vi "test.vi"() -> ()   [LabVIEW 2019]
uses:
  Valve_class/Valve.lvclass
panel:
  out "error out":errorcluster
  in  "VISA resource name":refnum<visa-resource-name>
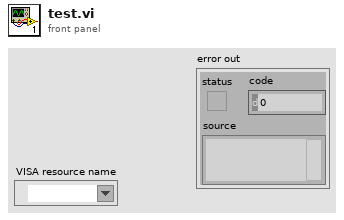
[diagram p1: front panel]
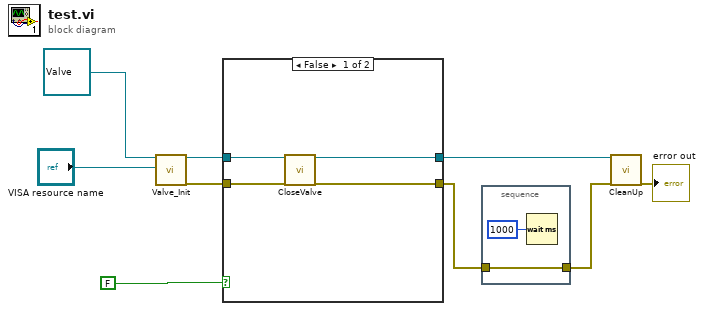
[diagram p0: block diagram]
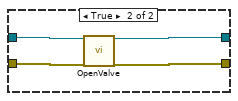
[diagram p2: hidden frame]
diagram:
  n1 = call "Valve_Init.vi"("object in"=refnum<class "Valve.lvclass"> refnum, "VISA resource name"="VISA resource name") -> ("object out"=w9:refnum<class "Valve.lvclass">, "error out"=w8:errorcluster)  [unwired: 16 in]
  n2 = case shown="False" FALSE {
    tunnel: w9 -> [w13 w17]
    tunnel: w8 -> [w11 w16]
    tunnel: [w12 w15] -> w5
    tunnel: [w10 w14] -> w4
    frame False {
      n3 = call-dynamic "CloseValve.vi"("object in"=w13, "error in (no error)"=w11) -> ("object out"=w12:refnum<class "Valve.lvclass">, "error out"=w10:errorcluster)  [unwired: 16 in]
    }
    frame True {
      n4 = call-dynamic "OpenValve.vi"("object in"=w17, "error in (no error)"=w16) -> ("object out"=w15:refnum<class "Valve.lvclass">, "error out"=w14:errorcluster)  [unwired: 16 in]
    }
  }
  n5 = stacked-sequence {
    tunnel: w4 -> [w18]
    tunnel: [w18] -> w3
    frame #0 {
      n6 = Wait (ms)(milliseconds to wait=u32 1000) -> ()  [unwired: 1 out]
    }
  }
  n7 = call-dynamic "CleanUp.vi"("object in"=w5, "error in (no error)"=w3) -> ("error out"=→"error out":errorcluster)  [unwired: 16 in, 1 out]
